vi "write to shutter line.vi"(8 "error in (no error)":errorcluster, 10 "Output Array":bool[](array[boolean])=[FALSE, FALSE, FALSE, FALSE, FALSE, FALSE, FALSE, FALSE], 11 "Waveform in":refnum<class "Waveform.lvclass">) -> (0 "error out":errorcluster, 3 "Waveform out":refnum<class "Waveform.lvclass">)   [LabVIEW 2012, in "Waveform.lvclass"]
uses:
  Waveform.lvclass
  Waveform.lvclass/Waveform.ctl
  <vilib>/DAQmx/write.llb/DAQmx Write (Digital 1D Bool 1Chan 1Samp).vi
  <vilib>/DAQmx/miscellaneous.llb/DAQmx Fill In Error Info.vi
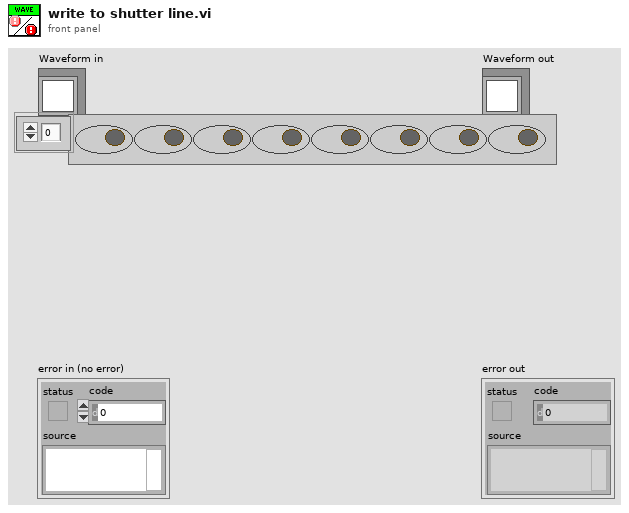
[diagram p1: front panel]
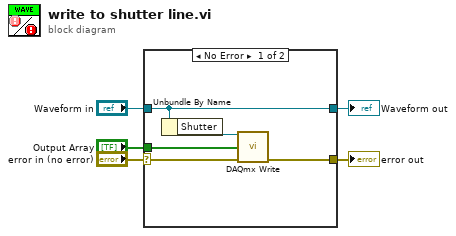
[diagram p0: block diagram]
diagram:
  n1 = case shown="No Error" "error in (no error)" {
    selector: "error in (no error)" -> [w8 w12]
    tunnel: [w7 w12] -> w4
    tunnel: [w10 w11] -> w2
    tunnel: "Waveform in" -> [w10 w11]
    tunnel: "Output Array" -> [w6 _]
    frame No Error {
      n2 = Unbundle By Name(w10) -> ("Shutter"=w9:refnum<k21>)
      n3 = call-poly <vilib>:"DAQmx Write.vi"("task/channels in"=w9, "data"=w6, "error in"=w8) -> ("error out"=w7:errorcluster)  [unwired: 10 in, 2 out]
    }
    frame Error {
    }
  }
  "error out" <- w4
  "Waveform out" <- w2
